vi "Stop Core.vi"(10 "final error code":i32, 11 "Water Level in":refnum<class "Water Level.lvclass">) -> (3 "Water Level out":refnum<class "Water Level.lvclass">)   [LabVIEW 2012, in "Water Level.lvclass"]
doc: "In override VIs of Stop Core.vi, an actor should invoke any code needed to stop all the parallel processes that it created during its run. This includes any nested actors that it created and any other asynchronously running VIs, such as a Time-Delated Message. It may also include all parallel loops in its Actor Core, although it is acceptable to stop those using a local signal on the Actor Core block diagram that is raised after the Call Parent Node finishes. \n\nThe <b>final error code</b> input tells the actor what error was set when this actor quit. Zero means there was no error. You can use this to decide whether this should be treated as a Normal Stop or an Emergency Stop for the purposes of signaling other actors. In general, any non-zero value should be treated as an Emergency Stop, though a given actor is free to choose other policies. Note that the particular error code 1608 indicates that this actor was itself stopped by an Emergency Stop and should pass that along."
uses:
  Water Level.lvclass
  Level Controller/Level Controller/Level Controller.lvclass
  Simulation/Simulation Data_Global.vi
  Simulation/Simulation.lvlib
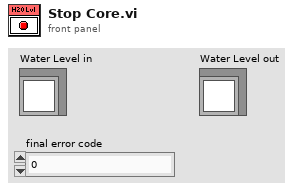
[diagram p1: front panel]
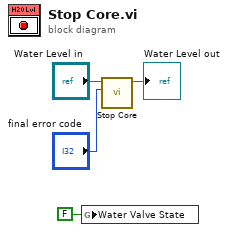
[diagram p0: block diagram]
diagram:
  n1 = global write "Simulation Data_Global.vi" "Water Valve State"(FALSE ("Water Valve State")) -> ()
  n2 = call-parent "Stop Core.vi"("final error code"="final error code", "Actor in"="Water Level in") -> ("Actor out"=→"Water Level out":refnum<class "Water Level.lvclass">)  [unwired: 9 in]
